vi "_PC_Daemon_Config_D999.vi"(8 "error in (no error)":errorcluster) -> (0 "error out":errorcluster)   [LabVIEW 2018]
uses:
  PublicSubVI/Ctl/RegistyFunc.ctl
  <resource>/objmgr/ni.var.rc
  <vilib>/Utility/miscctls.llb/LVBoundsTypeDef.ctl
panel:
  in  "Load":bool
  in  "Save":bool
  in  "Multiply":dbl[](array[numeric])=[1.0, 1.0, 1.0, 1.0, 1.0, 1.0, 1.0, 1.0, 1.0, 1.0, 1.0, 1.0]
  in  "Add":dbl[](array[numeric])=[0.0, 0.0, 0.0, 0.0, 0.0, 0.0, 0.0, 0.0, 0.0, 0.0, 0.0, 0.0]
  in  "Label":string[](array[string])=["", "", "", "", "", "", "", "", "", "", "", ""]
  in  "AI":string[](array[string])=["AI 0", "AI 1", "AI 2", "AI 3", "AI 4", "AI 5", "AI 6", "AI 7", "AI 8", "AI 9", "AI 10", "AI 11"]
  in  "AO":string[](array[string])=["AO 0", "AO 1", "AO 2", "AO 3", "AO 4", "AO 5", "AO 6", "AO 7", "AO 8"]
  in  "WriteValue":i16[](array[numeric])=[0, 0, 0, 0, 0, 0, 0, 0, 0] min=-4095 max=4095 step=1000
  in  "WriteColor":u32[](array[colorbox])=[16777224, 16777224, 16777224, 16777224, 16777224, 16777224, 16777224, 16777224, 16777224]
  in  "Scale":u16=1 min=1
  in  "Enable":bool
  in  "CEM(AO1)":bool
  in  "DYNODE(AO 0)":bool
  in  "ESPY(AO2)":bool
  in  "LENS(AO 3 : AO 8)":bool
  in  "Description":string="LENS : OFF; ESPY : OFF; DYNODE : OFF; CEN : OFF; "
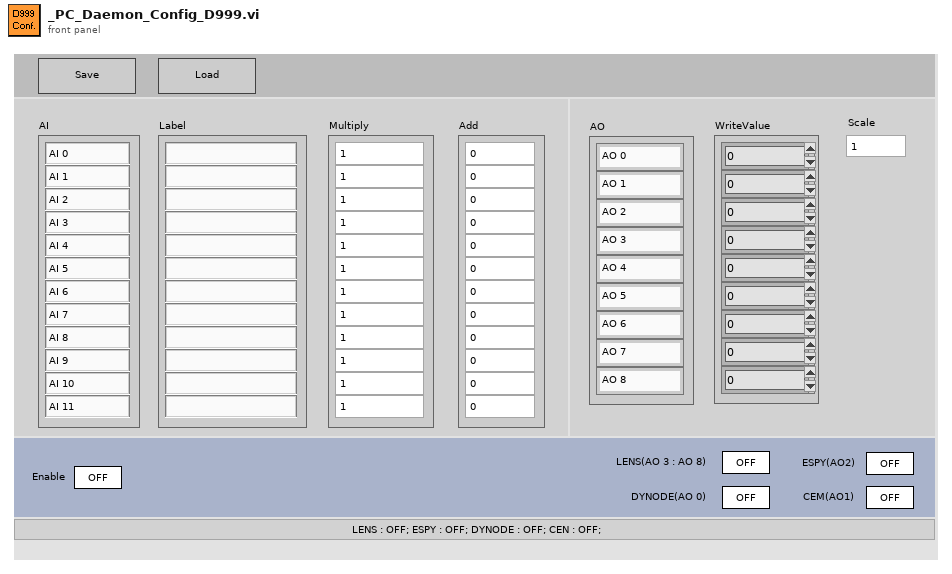
[diagram p1: front panel]
types:
  T1 = cluster{"Enable":refnum<vi>, "Label":refnum<vi>, "Multiply":refnum<vi>, "Add":refnum<vi>, "WriteColor":refnum<vi>, "WriteValue":refnum<vi>, "Description":refnum<vi>, "switch array":refnum<vi>[]}
  T2 = enum8{"Enabled", "Disabled", "Disabled and Grayed Out"}
  T3 = enum32{"Invalid", "Default", "Floating", "Floating/Auto-Hide", "Modal"}
  T4 = typedef "LVBoundsTypeDef.ctl" = cluster{"Width":u32, "Height":u32}
  T5 = cluster{"Label":string, "MultiValue":dbl, "AddValue":dbl}
  T6 = typedef "_ctl_RT_D999_Param.ctl" = cluster{"Enable":bool, "AI":cluster{"Label":string, "MultiValue":dbl, "AddValue":dbl}[], "AO":i16[], "Switch":bool[]}
  T7 = typedef "RegistyFunc.ctl" = enum16{"None", "FileAutoSave", "FileNoise", "FileSN", "ExeStatu", "WorkFolderPath", "MethodPath", "AVGItem", "LoopItem", "AutoRun", "BGColor", "LineColor", "LineWidth", "XGrid", "YGrid", "DeviceRefnum"}
  T8 = cluster{"Label":string[], "Multiply":dbl[], "Add":dbl[], "WriteValue":i16[], "switch":u32}
  T9 = typedef "eventvkey.ctl" = enum16{"ASCII", "Enter", "Return", "Shift", "Ctrl", "Alt", "Cmd", "Opt", "Caps", "NumLock", "Clear", "Break", "Up", "Down", "Left", "Right", "Insert", "Delete", "Home", "End", "PageUp", "PageDown", "Escape", "Help", "Pause", "ScrollLock", "F1", "F2", "F3", "F4", "F5", "F6", "F7", "F8", "F9", "F10", "F11", "F12", "F13", "F14", "F15", "F16", "F17", "F18", "F19", "F20", "F21", "F22", "F23", "F24", "Play", "VolumeUp", "VolumeDown", "Mute", "Two Byte Char"}
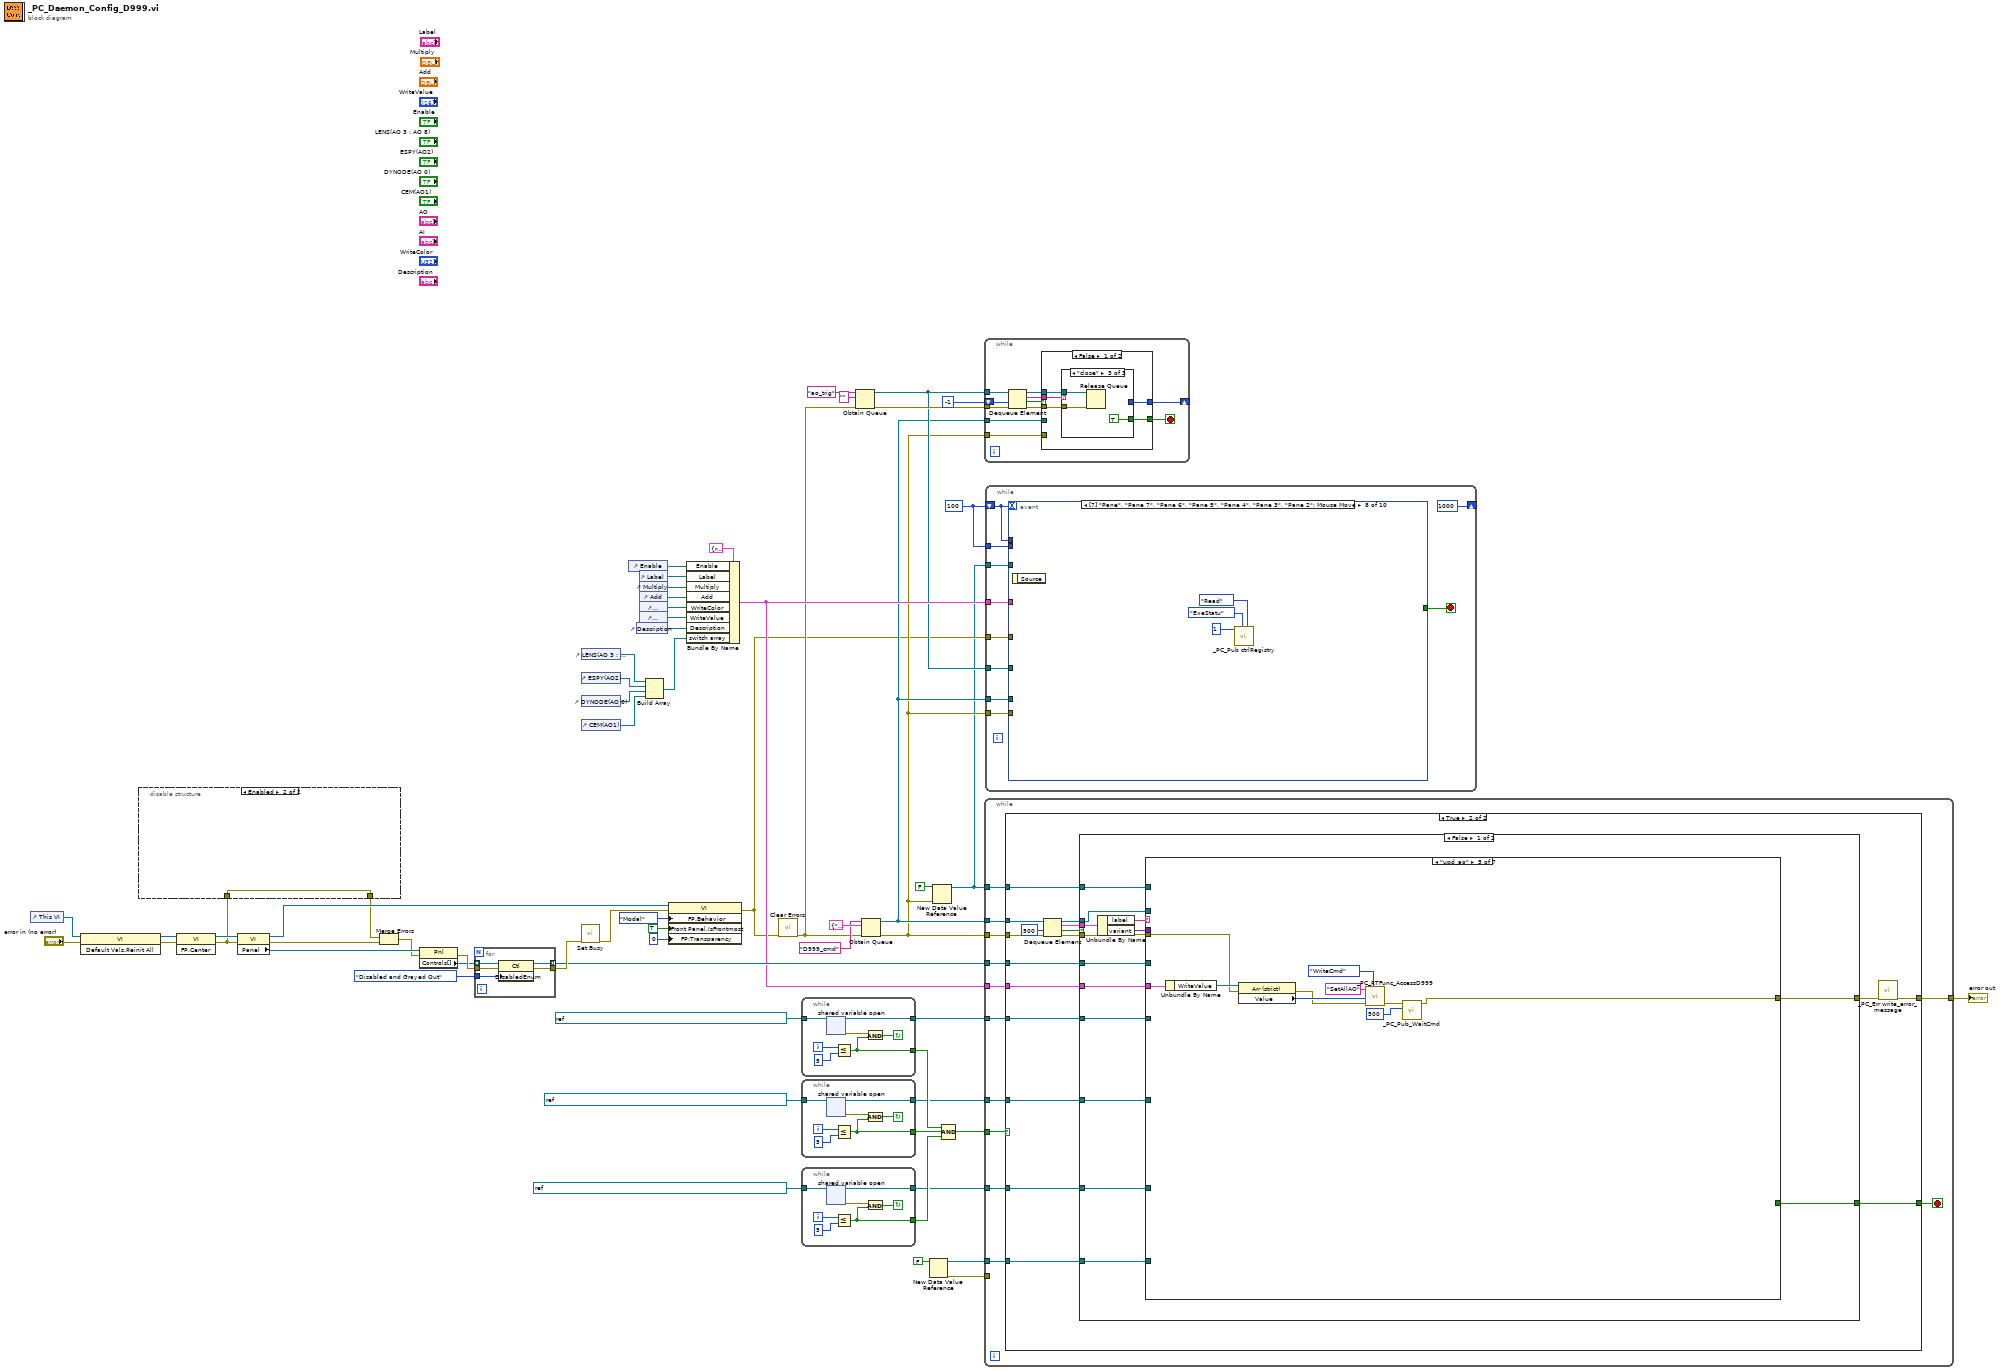
[diagram p0: block diagram]
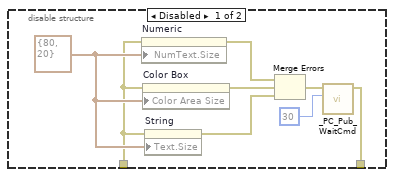
[diagram p2: hidden frame]
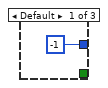
[diagram p3: hidden frame]
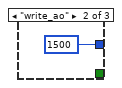
[diagram p4: hidden frame]
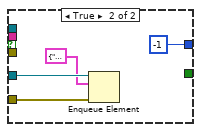
[diagram p5: hidden frame]
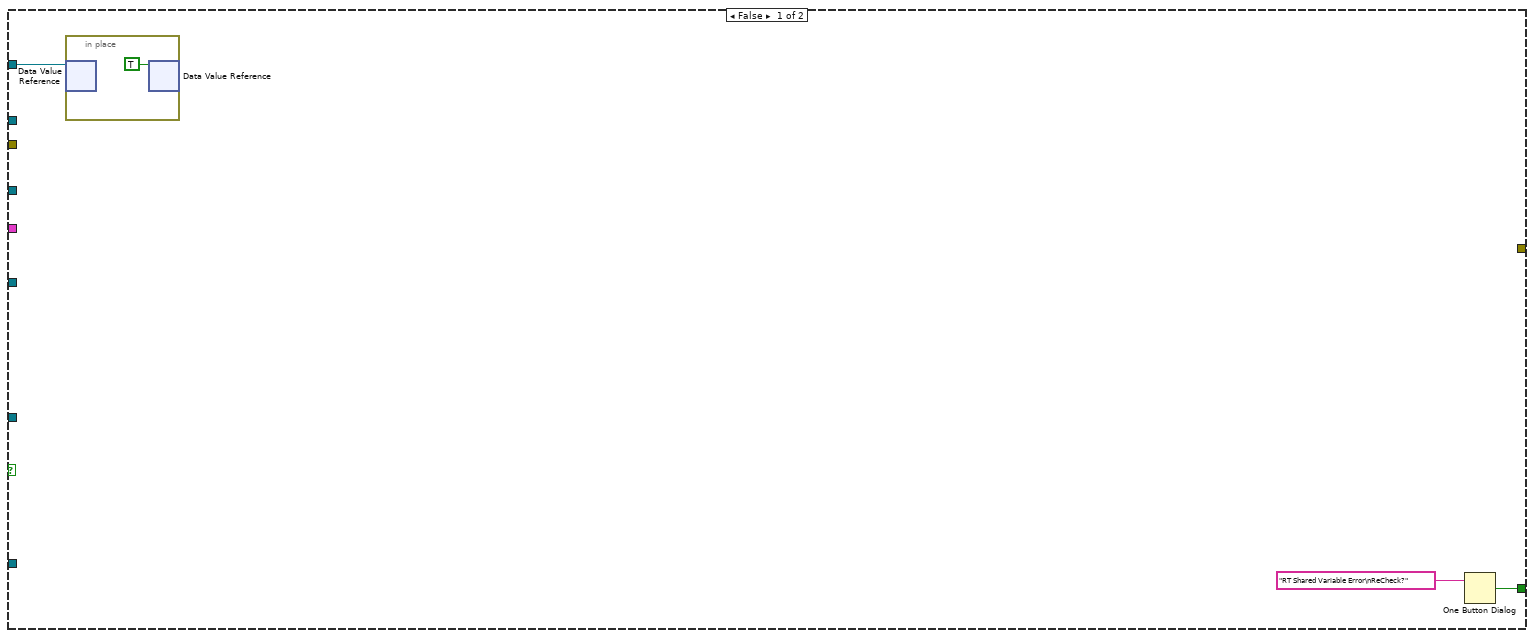
[diagram p6: hidden frame]
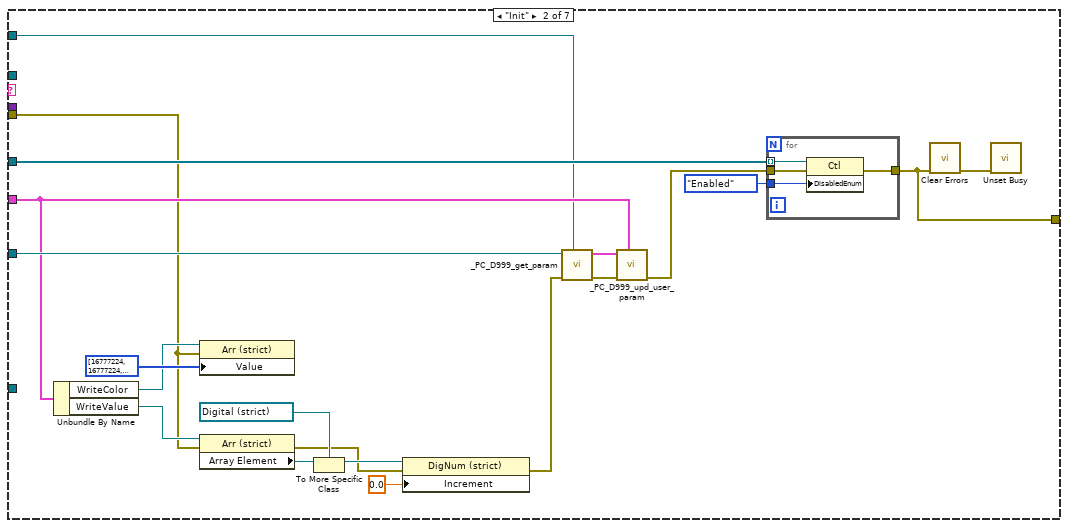
[diagram p8: hidden frame]
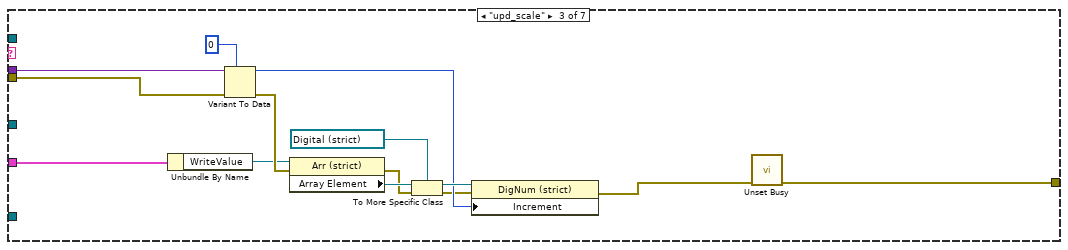
[diagram p9: hidden frame]
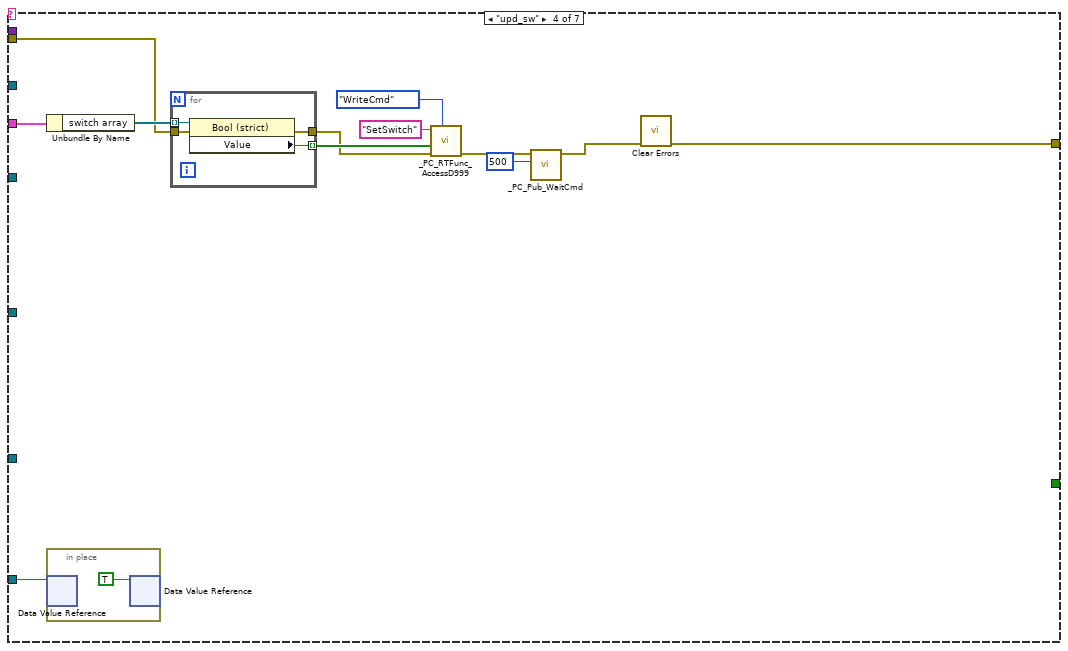
[diagram p10: hidden frame]
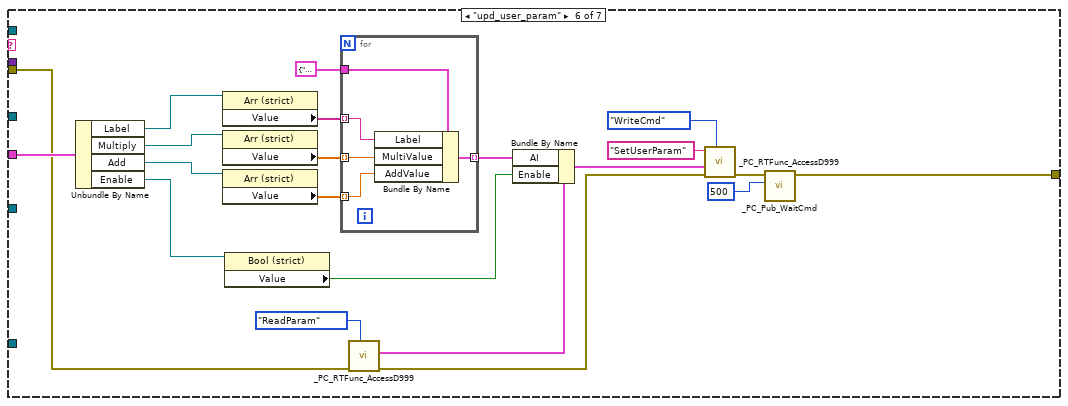
[diagram p11: hidden frame]
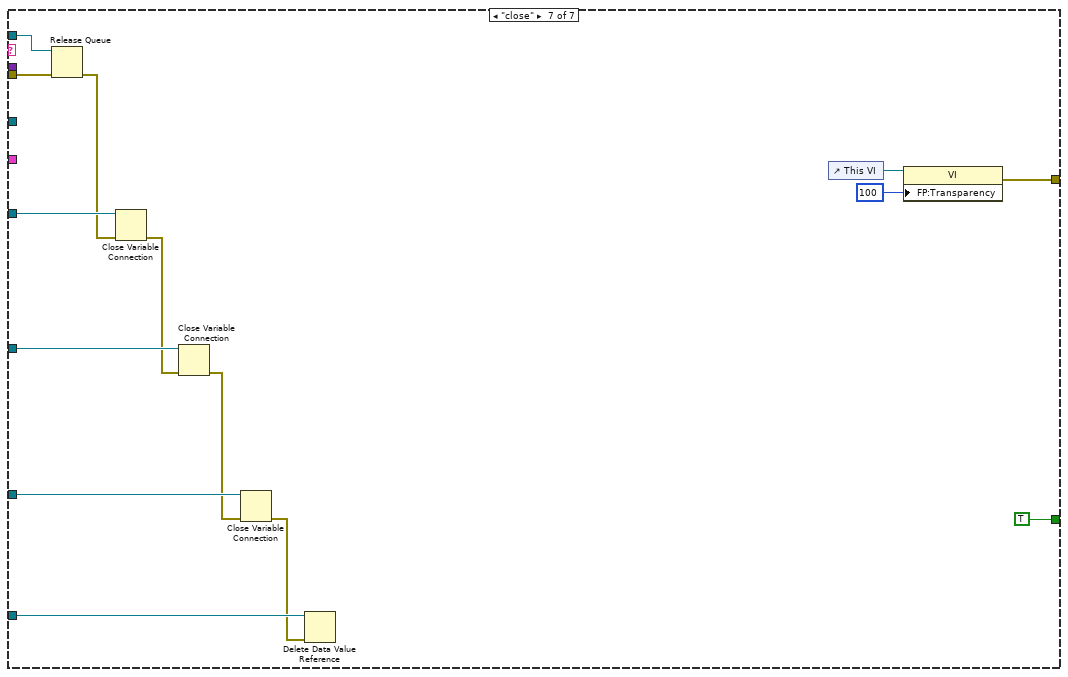
[diagram p12: hidden frame]
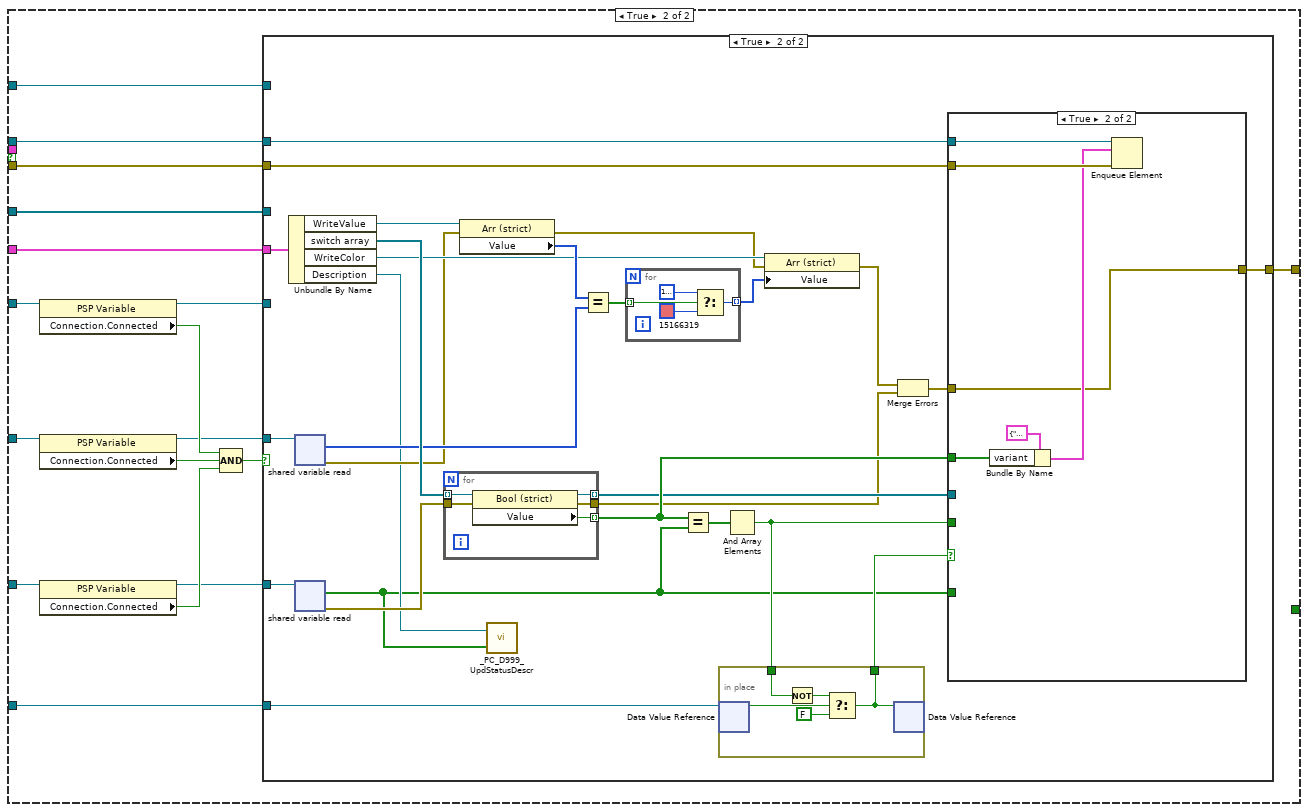
[diagram p13: hidden frame]
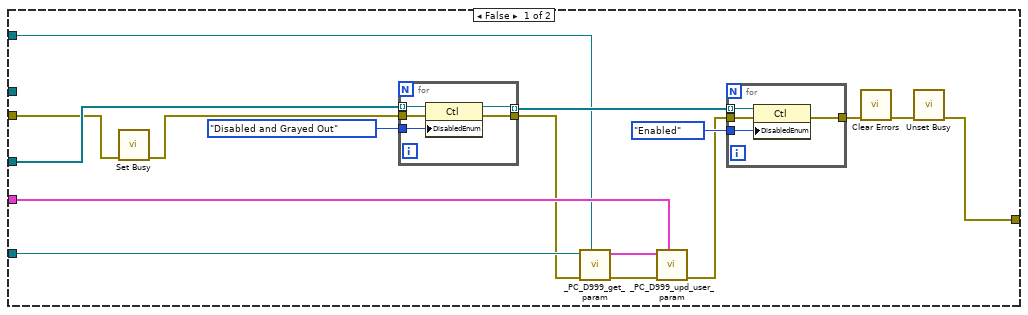
[diagram p14: hidden frame]
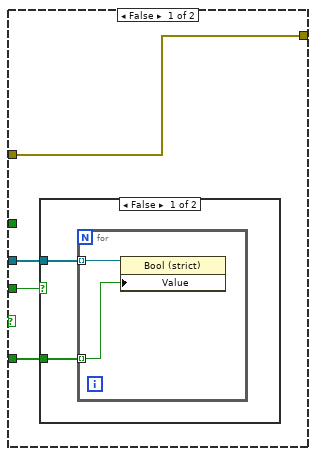
[diagram p15: hidden frame]
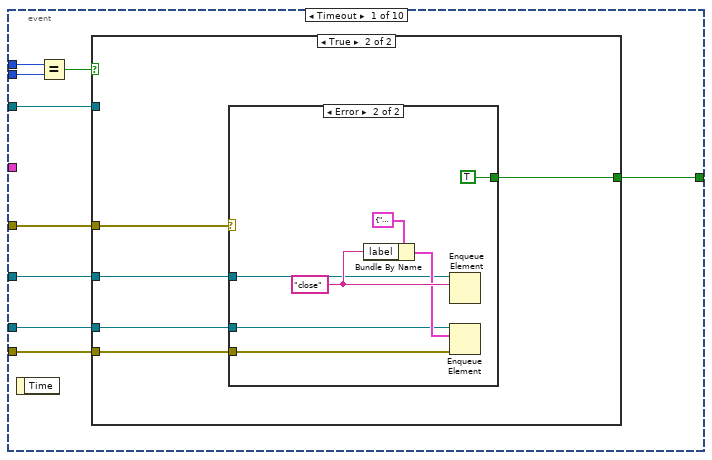
[diagram p17: hidden frame]
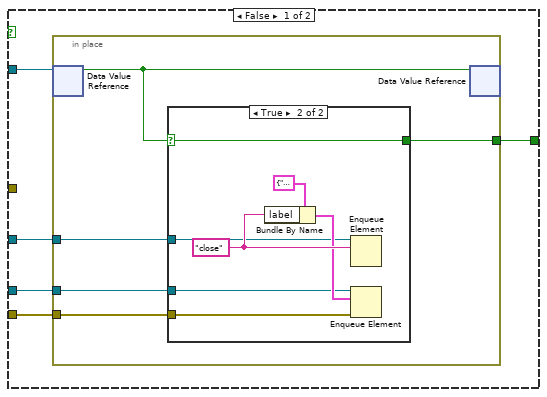
[diagram p18: hidden frame]
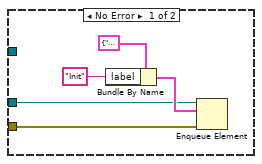
[diagram p20: hidden frame]
diagram:
  w2 = 100
  n1 = control-ref of="This VI"() -> (w59:refnum<vi>)
  n2 = invoke class="VI" method="Default Vals.Reinit All"(reference=w59, error in="error in (no error)") -> (reference out=w60:refnum<vi>, error out=w57:errorcluster)  [unwired: 1 in, 1 out]
  n3 = invoke class="VI" method="FP.Center"(reference=w60, error in=w57) -> (reference out=w52:refnum<vi>, error out=w9:errorcluster)  [unwired: 1 in, 1 out]
  n4 = disable-structure shown="Enabled" {
    disable-tunnel: w9 -> [w64 w71]
    disable-tunnel: [w63 w71] -> w6
    frame Disabled {
      w70 = T4 {"Width"=80, "Height"=20} ("Numeric Text.Size")
      n5 = property on="Numeric" class="DigNum (strict)"(error in=w64, "NumText.Size"=w70) -> (error out=w69:errorcluster)  [unwired: 1 in, 1 out]
      n6 = property on="Color Box" class="ColBox"(error in=w64, "Color Area Size"=w70) -> (error out=w68:errorcluster)  [unwired: 1 in, 1 out]
      n7 = property on="String" class="Str"(error in=w64, "Text.Size"=w70) -> (error out=w67:errorcluster)  [unwired: 1 in, 1 out]
      n8 = Merge Errors(w69, w68, w67) -> (w65:errorcluster)
      n9 = call "_PC_Pub_WaitCmd.vi"("milliseconds to wait"=u32 30, "error in (no error)"=w65) -> ("error out"=w63:errorcluster)  [unwired: 9 in]
    }
    frame Enabled {
    }
  }
  n10 = property class="VI"(reference=w52, error in=w9) -> (reference out=w51:refnum<vi>, error out=w7:errorcluster, "Panel"=w58:refnum<vi>)
  n11 = Merge Errors(w6, w7) -> (w5:errorcluster)
  n12 = property class="Pnl"(reference=w58, error in=w5) -> (error out=w55:errorcluster, "Controls[]"=w54:refnum<vi>[])  [unwired: 1 out]
  n13 = for {
    tunnel: w54 -> [w76] mode=indexing
    tunnel: T2."Disabled and Grayed Out" ("Disabled") -> [w75]
    tunnel: [w74] -> w23 mode=indexing
    tunnel: [w73] -> w50
    tunnel: w55 -> [w72]
    n14 = property class="Ctl"(reference=w76, error in=w72, "DisabledEnum"=w75) -> (reference out=w74:refnum<vi>, error out=w73:errorcluster)
  }
  n15 = control-ref of="LENS(AO 3 : AO 8)"() -> (w34:refnum<vi>)
  n16 = control-ref of="ESPY(AO2)"() -> (w35:refnum<vi>)
  n17 = control-ref of="DYNODE(AO 0)"() -> (w36:refnum<vi>)
  n18 = control-ref of="CEM(AO1)"() -> (w37:refnum<vi>)
  n19 = call <vilib>:"Set Busy.vi"("error in (no error)"=w50) -> ("error out"=w8:errorcluster)  [unwired: 9 in, 1 out]
  n20 = control-ref of="Enable"() -> (w32:refnum<vi>)
  n21 = control-ref of="Description"() -> (w26:refnum<vi>)
  n22 = control-ref of="Label"() -> (w31:refnum<vi>)
  n23 = control-ref of="Multiply"() -> (w30:refnum<vi>)
  n24 = control-ref of="Add"() -> (w29:refnum<vi>)
  n25 = control-ref of="WriteColor"() -> (w28:refnum<vi>)
  n26 = control-ref of="WriteValue"() -> (w27:refnum<vi>)
  n27 = Build Array(w34, w35, w36, w37) -> (w25:refnum<vi>[])
  n28 = property class="VI"(reference=w51, error in=w8, "FP.Behavior"=T3."Modal" ("Front Panel Window:Behavior"), "Front Panel.IsFrontmost"=TRUE ("Front Panel Window:Is Frontmost"), "FP:Transparency"=u8 0 ("Front Panel Window:Transparency")) -> (error out=w4:errorcluster)  [unwired: 1 out]
  n29 = Bundle By Name(cluster=T1 {"Enable"=refnum, "Label"=refnum, "Multiply"=refnum, "Add"=refnum, "WriteColor"=refnum, "WriteValue"=refnum, "Description"=refnum, "switch array"=[]}, "Enable"=w32, "Label"=w31, "Multiply"=w30, "Add"=w29, "WriteColor"=w28, "WriteValue"=w27, "Description"=w26, "switch array"=w25) -> (w20:T1)
  n30 = call <vilib>:"Clear Errors.vi"("error in (no error)"=w4) -> ("error out"=w17:errorcluster)  [unwired: 5 in, 1 out]
  n31 = while {
    tunnel: [w77] -> w45
    tunnel: refnum<k21> "ni.var.psp://NI-sbRIO/_RT_CtrlLoop_D999_Variables/D999_Exist" ("shared variable refnum in") -> [w83]
    tunnel: [w82] -> w46
    i -> [w80]
    stop <- w78 continue-if-true
    n32 = shared-variable-open(w83) -> (w82:refnum<k21>, w79:errorcluster)  [unwired: 1 in]
    n33 = Less Or Equal?(x=w80, y=5) -> (x <= y?=w77:bool)
    n34 = And(x=w79, y=w77) -> (x .and. y?=w78:bool)
  }
  n35 = while {
    tunnel: [w84] -> w44
    tunnel: refnum<k21> "ni.var.psp://NI-sbRIO/_RT_CtrlLoop_D999_Variables/D999_AO_Res" ("shared variable refnum in") -> [w90]
    tunnel: [w89] -> w39
    i -> [w87]
    stop <- w85 continue-if-true
    n36 = shared-variable-open(w90) -> (w89:refnum<k21>, w86:errorcluster)  [unwired: 1 in]
    n37 = Less Or Equal?(x=w87, y=5) -> (x <= y?=w84:bool)
    n38 = And(x=w86, y=w84) -> (x .and. y?=w85:bool)
  }
  n39 = while {
    tunnel: [w91] -> w43
    tunnel: refnum<k21> "ni.var.psp://NI-sbRIO/_RT_CtrlLoop_D999_Variables/D999_Switch_Res" ("shared variable refnum in") -> [w97]
    tunnel: [w96] -> w38
    i -> [w94]
    stop <- w92 continue-if-true
    n40 = shared-variable-open(w97) -> (w96:refnum<k21>, w93:errorcluster)  [unwired: 1 in]
    n41 = Less Or Equal?(x=w94, y=5) -> (x <= y?=w91:bool)
    n42 = And(x=w93, y=w91) -> (x .and. y?=w92:bool)
  }
  n43 = Obtain Queue(name (unnamed)="ao_trig", element data type="", error in (no error)=w17) -> (queue out=w16:refnum<queue>, error out=w18:errorcluster)  [unwired: 2 in, 1 out]
  n44 = Obtain Queue(name (unnamed)="D999_cmd", element data type=cluster{"label":string, "variant":variant} {"label"="", "variant"=variant}, error in (no error)=w17) -> (queue out=w13:refnum<queue>, error out=w10:errorcluster)  [unwired: 2 in, 1 out]
  n45 = New Data Value Reference(data value=FALSE) -> (data value reference=w24:refnum<data-value>, error out=w21:errorcluster)  [unwired: 1 in]
  n46 = New Data Value Reference(data value=FALSE, error in=w10) -> (data value reference=w1:refnum<data-value>)  [unwired: 1 out]
  n47 = Compound Arithmetic op=AND(w45, w44, w43) -> (w42:bool)
  n48 = while {
    tunnel: w16 -> [w108]
    tunnel: w18 -> [w106]
    shift-right: [w101] -> _
    shift-left: -1 ("timeout in ms (-1)") -> [w107]
    tunnel: w13 -> [w99]
    tunnel: w10 -> [w98]
    stop <- w100 stop-if-true
    n49 = Dequeue Element(queue=w108, timeout in ms (-1)=w107, error in (no error)=w106) -> (queue out=w102:refnum<queue>, element=w104:string, timed out?=w105:bool, error out=w103:errorcluster)
    n50 = case shown="False" w105 {
      tunnel: w104 -> [w113 _]
      tunnel: w103 -> [w112 _]
      tunnel: w102 -> [w109 _]
      tunnel: [w111 -1] -> w101
      tunnel: [w110 _] -> w100
      tunnel: w99 -> [_ w121]
      tunnel: w98 -> [_ w120]
      frame False {
        n51 = case shown="\"close\"" w113 {
          tunnel: w112 -> [_ _ w116]
          tunnel: [-1 1500 _] -> w111
          tunnel: [_ _ TRUE] -> w110
          tunnel: w109 -> [_ _ w117]
          frame Default {
          }
          frame "write_ao" {
          }
          frame "close" {
            n52 = Release Queue(queue=w117, error in (no error)=w116) -> ()  [unwired: 1 in, 3 out]
          }
        }
      }
      frame True {
        n53 = Enqueue Element(queue=w121, element=cluster{"label":string, "variant":variant} {"label"="upd_ao", "variant"=variant}, error in (no error)=w120) -> ()  [unwired: 1 in, 3 out]
      }
    }
  }
  n54 = while {
    tunnel: w13 -> [w134]
    tunnel: w10 -> [w133]
    tunnel: w46 -> [w132]
    tunnel: w42 -> [w130]
    tunnel: w39 -> [w129]
    tunnel: w38 -> [w128]
    tunnel: w20 -> [w127]
    tunnel: w24 -> [w126]
    tunnel: w23 -> [w125]
    tunnel: w21 -> [_]
    tunnel: [w124] -> w12
    tunnel: w1 -> [w123]
    stop <- w131 stop-if-true
    n55 = case shown="True" w130 {
      tunnel: w134 -> [_ w155]
      tunnel: w133 -> [_ w154]
      tunnel: w132 -> [_ w149]
      tunnel: [w136 w141] -> w131
      tunnel: w129 -> [_ w148]
      tunnel: w128 -> [_ w147]
      tunnel: w127 -> [_ w146]
      tunnel: w126 -> [_ w144]
      tunnel: w125 -> [_ w143]
      tunnel: [_ w140] -> w124
      tunnel: w123 -> [w135 w139]
      frame False {
        n56 = in-place {
          n57 = in-place-dvr #1(w135) -> ()  [unwired: 2 out]
          n58 = in-place-dvr #1(TRUE ("data value")) -> ()  [unwired: 2 out]
        }
        n59 = One Button Dialog(message="RT Shared Variable Error\nReCheck?") -> (true=w136:bool)  [unwired: 1 in]
      }
      frame True {
        n60 = Dequeue Element(queue=w155, timeout in ms (-1)=500, error in (no error)=w154) -> (queue out=w145:refnum<queue>, element=w150:cluster{"label":string, "variant":variant}, timed out?=w152:bool, error out=w151:errorcluster)
        n61 = case shown="False" w152 {
          tunnel: w151 -> [w161 w281]
          tunnel: w150 -> [w169 _]
          tunnel: w149 -> [w166 w292]
          tunnel: w148 -> [w165 w291]
          tunnel: w147 -> [w164 w290]
          tunnel: w146 -> [w162 w283]
          tunnel: w145 -> [w157 w282]
          tunnel: w144 -> [w160 w280]
          tunnel: w143 -> [w163 w278]
          tunnel: [w159 w277] -> w142
          tunnel: [w158 _] -> w141
          tunnel: w139 -> [w156 w276]
          frame False {
            n62 = Unbundle By Name(w169) -> ("label"=w168:string, "variant"=w167:variant)
            n63 = case shown="\"upd_ao\"" w168 {
              tunnel: w167 -> [_ _ w203 _ _ _ _]
              tunnel: w166 -> [_ w187 _ _ _ _ w272]
              tunnel: w165 -> [_ _ _ _ _ _ w270]
              tunnel: w164 -> [_ _ _ _ _ _ w268]
              tunnel: w163 -> [_ w190 _ _ _ _ _]
              tunnel: w162 -> [_ w183 w199 w215 w230 w244 _]
              tunnel: w161 -> [w170 w174 w195 w210 w228 w237 w273]
              tunnel: w160 -> [_ _ _ w212 _ _ w269]
              tunnel: [w170 w172 w196 w209 w226 w236 w262] -> w159
              tunnel: [_ _ _ _ _ _ TRUE] -> w158
              tunnel: w157 -> [_ _ _ _ _ _ w274]
              tunnel: w156 -> [_ w171 _ _ _ _ _]
              frame Default {
              }
              frame "Init" {
                n64 = Unbundle By Name(w183) -> ("WriteColor"=w175:refnum<vi>, "WriteValue"=w177:refnum<vi>)
                n65 = property class="Arr (strict)"(reference=w175, error in=w174, "Value"=u32[] [16777224, 16777224, 16777224, 16777224, 16777224, 16777224, 16777224, 16777224, 16777224]) -> ()  [unwired: 2 out]
                n66 = property class="Arr (strict)"(reference=w177, error in=w174) -> (error out=w178:errorcluster, "Array Element"=w182:refnum<vi>)  [unwired: 1 out]
                n67 = To More Specific Class(target class=refnum<vi> refnum ("Numeric"), reference=w182) -> (specific class reference=w179:refnum<vi>)  [unwired: 1 in, 1 out]
                n68 = property class="DigNum (strict)"(reference=w179, error in=w178, "Increment"=0.0 ("Data Entry Limits:Increment")) -> (error out=w173:errorcluster)  [unwired: 1 out]
                n69 = call "_PC_D999_get_param.vi"("stop cmd"=w171, "error in (no error)"=w173, "D999_exist SV"=w187) -> ("error out"=w188:errorcluster, "D999_Param"=w189:T6)  [unwired: 7 in]
                n70 = call "_PC_D999_upd_user_param.vi"("refnum cluster"=w183, "error in (no error)"=w188, "D999_Param"=w189) -> ("error out"=w186:errorcluster)  [unwired: 8 in]
                n71 = for {
                  tunnel: w190 -> [w194] mode=indexing
                  tunnel: T2."Enabled" ("Disabled") -> [w193]
                  tunnel: [w192] -> w172
                  tunnel: w186 -> [w191]
                  n72 = property class="Ctl"(reference=w194, error in=w191, "DisabledEnum"=w193) -> (error out=w192:errorcluster)  [unwired: 1 out]
                }
                n73 = call <vilib>:"Clear Errors.vi"("error in (no error)"=w172) -> ("error out"=w184:errorcluster)  [unwired: 5 in, 1 out]
                n74 = call <vilib>:"Unset Busy.vi"("error in (no error)"=w184) -> ()  [unwired: 10 in, 1 out]
              }
              frame "upd_scale" {
                n75 = Unbundle By Name(w199) -> ("WriteValue"=w198:refnum<vi>)
                n76 = Variant To Data(error in=w195, type=u16 0 ("NewVal"), Variant=w203) -> (data=w204:u16, error out=w200:errorcluster)
                n77 = property class="Arr (strict)"(reference=w198, error in=w200) -> (error out=w202:errorcluster, "Array Element"=w207:refnum<vi>)  [unwired: 1 out]
                n78 = To More Specific Class(target class=refnum<vi> refnum ("Numeric"), reference=w207, error in=w202) -> (specific class reference=w206:refnum<vi>, error out=w201:errorcluster)
                n79 = property class="DigNum (strict)"(reference=w206, error in=w201, "Increment"=w204) -> (error out=w197:errorcluster)  [unwired: 1 out]
                n80 = call <vilib>:"Unset Busy.vi"("error in (no error)"=w197) -> ("error out"=w196:errorcluster)  [unwired: 10 in]
              }
              frame "upd_sw" {
                n81 = Unbundle By Name(w215) -> ("switch array"=w214:refnum<vi>[])
                n82 = in-place {
                  n83 = in-place-dvr #2(w212) -> ()  [unwired: 2 out]
                  n84 = in-place-dvr #2(TRUE ("data value")) -> ()  [unwired: 2 out]
                }
                n85 = for {
                  tunnel: w214 -> [w225] mode=indexing
                  tunnel: [w224] -> w219 mode=indexing
                  tunnel: w210 -> [w223]
                  tunnel: [w222] -> w213
                  n86 = property class="Bool (strict)"(reference=w225, error in=w223) -> (error out=w222:errorcluster, "Value"=w224:bool)  [unwired: 1 out]
                }
                n87 = call "_PC_RTFunc_AccessD999.vi"("Function"=enum16{"WriteCmd", "ReadParam", "ReadResponse"}."WriteCmd", "error in (no error)"=w213, "Variant"=w219, "Cmd"="SetSwitch") -> ("error out"=w218:errorcluster)  [unwired: 6 in, 1 out]
                n88 = call "_PC_Pub_WaitCmd.vi"("milliseconds to wait"=u32 500, "error in (no error)"=w218) -> ("error out"=w211:errorcluster)  [unwired: 9 in]
                n89 = call <vilib>:"Clear Errors.vi"("error in (no error)"=w211) -> ("error out"=w209:errorcluster)  [unwired: 5 in, 1 out]
              }
              frame "upd_ao" {
                n90 = Unbundle By Name(w230) -> ("WriteValue"=w229:refnum<vi>)
                n91 = property class="Arr (strict)"(reference=w229, error in=w228) -> (error out=w227:errorcluster, "Value"=w234:i16[])  [unwired: 1 out]
                n92 = call "_PC_RTFunc_AccessD999.vi"("Function"=enum16{"WriteCmd", "ReadParam", "ReadResponse"}."WriteCmd", "error in (no error)"=w227, "Variant"=w234, "Cmd"="SetAllAO") -> ("error out"=w233:errorcluster)  [unwired: 6 in, 1 out]
                n93 = call "_PC_Pub_WaitCmd.vi"("milliseconds to wait"=u32 500, "error in (no error)"=w233) -> ("error out"=w226:errorcluster)  [unwired: 9 in]
              }
              frame "upd_user_param" {
                n94 = Unbundle By Name(w244) -> ("Label"=w243:refnum<vi>, "Multiply"=w242:refnum<vi>, "Add"=w241:refnum<vi>, "Enable"=w240:refnum<vi>)
                n95 = property class="Arr (strict)"(reference=w243) -> ("Value"=w253:string[])  [unwired: 1 in, 2 out]
                n96 = property class="Arr (strict)"(reference=w242) -> ("Value"=w252:dbl[])  [unwired: 1 in, 2 out]
                n97 = property class="Arr (strict)"(reference=w241) -> ("Value"=w251:dbl[])  [unwired: 1 in, 2 out]
                n98 = property class="Bool (strict)"(reference=w240) -> ("Value"=w248:bool)  [unwired: 1 in, 2 out]
                n99 = for {
                  tunnel: T5 {"Label"="", "MultiValue"=0.0, "AddValue"=0.0} ("EC_Param Cluster") -> [w261]
                  tunnel: w253 -> [w260] mode=indexing
                  tunnel: w252 -> [w259] mode=indexing
                  tunnel: w251 -> [w258] mode=indexing
                  tunnel: [w257] -> w250 mode=indexing
                  n100 = Bundle By Name(cluster=w261, "Label"=w260, "MultiValue"=w259, "AddValue"=w258) -> (w257:T5)
                }
                n101 = call "_PC_RTFunc_AccessD999.vi"("Function"=enum16{"WriteCmd", "ReadParam", "ReadResponse"}."ReadParam", "error in (no error)"=w237) -> ("error out"=w246:errorcluster, "D999_Param"=w249:T6)  [unwired: 8 in]
                n102 = Bundle By Name(cluster=w249, "AI"=w250, "Enable"=w248) -> (w247:T6)
                n103 = call "_PC_RTFunc_AccessD999.vi"("Function"=enum16{"WriteCmd", "ReadParam", "ReadResponse"}."WriteCmd", "error in (no error)"=w246, "Variant"=w247, "Cmd"="SetUserParam") -> ("error out"=w239:errorcluster)  [unwired: 6 in, 1 out]
                n104 = call "_PC_Pub_WaitCmd.vi"("milliseconds to wait"=u32 500, "error in (no error)"=w239) -> ("error out"=w236:errorcluster)  [unwired: 9 in]
              }
              frame "close" {
                n105 = Release Queue(queue=w274, error in (no error)=w273) -> (error out=w271:errorcluster)  [unwired: 1 in, 2 out]
                n106 = Close Variable Connection(8:w271, 11:w272) -> (0:w267:errorcluster)
                n107 = Close Variable Connection(8:w267, 11:w270) -> (0:w266:errorcluster)
                n108 = Close Variable Connection(8:w266, 11:w268) -> (0:w265:errorcluster)
                n109 = Delete Data Value Reference(data value reference=w269, error in=w265) -> ()  [unwired: 2 out]
                n110 = control-ref of="This VI"() -> (w264:refnum<vi>)
                n111 = property class="VI"(reference=w264, "FP:Transparency"=u8 100 ("Front Panel Window:Transparency")) -> (error out=w262:errorcluster)  [unwired: 1 in, 1 out]
              }
            }
          }
          frame True {
            n112 = property class="PSP Variable"(reference=w292) -> (reference out=w279:refnum<k21>, "Connection.Connected"=w288:bool)  [unwired: 1 in, 1 out]
            n113 = property class="PSP Variable"(reference=w291) -> (reference out=w285:refnum<k21>, "Connection.Connected"=w289:bool)  [unwired: 1 in, 1 out]
            n114 = property class="PSP Variable"(reference=w290) -> (reference out=w284:refnum<k21>, "Connection.Connected"=w287:bool)  [unwired: 1 in, 1 out]
            n115 = Compound Arithmetic op=AND(w288, w289, w287) -> (w286:bool)
            n116 = case shown="True" w286 {
              tunnel: w285 -> [_ w344]
              tunnel: w284 -> [_ w343]
              tunnel: w283 -> [w305 w342]
              tunnel: w282 -> [_ w327]
              tunnel: w281 -> [w296 w328]
              tunnel: w280 -> [_ w337]
              tunnel: w279 -> [w306 _]
              tunnel: w278 -> [w299 _]
              tunnel: [w294 w320] -> w277
              tunnel: w276 -> [w293 _]
              frame False {
                n117 = call <vilib>:"Set Busy.vi"("error in (no error)"=w296) -> ("error out"=w295:errorcluster)  [unwired: 9 in, 1 out]
                n118 = for {
                  tunnel: w299 -> [w313] mode=indexing
                  tunnel: T2."Disabled and Grayed Out" ("Disabled") -> [w312]
                  tunnel: [w311] -> w297
                  tunnel: w295 -> [w310]
                  tunnel: [w309] -> w298 mode=indexing
                  n119 = property class="Ctl"(reference=w313, error in=w310, "DisabledEnum"=w312) -> (reference out=w309:refnum<vi>, error out=w311:errorcluster)
                }
                n120 = call "_PC_D999_get_param.vi"("stop cmd"=w293, "error in (no error)"=w297, "D999_exist SV"=w306) -> ("error out"=w307:errorcluster, "D999_Param"=w308:T6)  [unwired: 7 in]
                n121 = call "_PC_D999_upd_user_param.vi"("refnum cluster"=w305, "error in (no error)"=w307, "D999_Param"=w308) -> ("error out"=w301:errorcluster)  [unwired: 8 in]
                n122 = for {
                  tunnel: w298 -> [w317] mode=indexing
                  tunnel: T2."Enabled" ("Disabled") -> [w316]
                  tunnel: [w315] -> w302
                  tunnel: w301 -> [w314]
                  n123 = property class="Ctl"(reference=w317, error in=w314, "DisabledEnum"=w316) -> (error out=w315:errorcluster)  [unwired: 1 out]
                }
                n124 = call <vilib>:"Clear Errors.vi"("error in (no error)"=w302) -> ("error out"=w303:errorcluster)  [unwired: 5 in, 1 out]
                n125 = call <vilib>:"Unset Busy.vi"("error in (no error)"=w303) -> ("error out"=w294:errorcluster)  [unwired: 10 in]
              }
              frame True {
                n126 = Unbundle By Name(w342) -> ("WriteValue"=w340:refnum<vi>, "switch array"=w341:refnum<vi>[], "WriteColor"=w330:refnum<vi>, "Description"=w319:refnum<vi>)
                n127 = shared-variable-read(w344) -> (w326:errorcluster, w339:i16[])  [unwired: 1 in, 1 out]
                n128 = shared-variable-read(w343) -> (w324:errorcluster, w318:bool[])  [unwired: 1 in, 1 out]
                n129 = for {
                  tunnel: w341 -> [w372] mode=indexing
                  tunnel: [w371] -> w335 mode=indexing
                  tunnel: [w370] -> w332 mode=indexing
                  tunnel: w324 -> [w369]
                  tunnel: [w368] -> w322
                  n130 = property class="Bool (strict)"(reference=w372, error in=w369) -> (reference out=w370:refnum<vi>, error out=w368:errorcluster, "Value"=w371:bool)
                }
                n131 = property class="Arr (strict)"(reference=w340, error in=w326) -> (error out=w325:errorcluster, "Value"=w334:i16[])  [unwired: 1 out]
                n132 = call "_PC_D999_UpdStatusDescr.vi"("Switch Enable"=w318, "Description"=w319) -> ()  [unwired: 1 in]
                n133 = Equal?(x=w334, y=w339) -> (x = y?=w329:bool[])
                n134 = for {
                  tunnel: w329 -> [w348] mode=indexing
                  tunnel: [w345] -> w331 mode=indexing
                  n135 = Select(t=u32 16777224, s=w348, f=u32 15166319) -> (s? t:f=w345:u32)
                }
                n136 = Equal?(x=w335, y=w318) -> (x = y?=w338:bool[])
                n137 = And Array Elements(Boolean array=w338) -> (logical AND=w333:bool)
                n138 = in-place {
                  in-place-border: w333 -> [w366]
                  in-place-border: [w363] -> w336
                  n139 = in-place-dvr #3(w337) -> (w367:bool)  [unwired: 1 out]
                  n140 = Not(x=w366) -> (.not. x?=w365:bool)
                  n141 = Select(t=w365, s=w367, f=FALSE) -> (s? t:f=w363:bool)
                  n142 = in-place-dvr #3(w363) -> ()  [unwired: 2 out]
                }
                n143 = property class="Arr (strict)"(reference=w330, error in=w325, "Value"=w331) -> (error out=w323:errorcluster)  [unwired: 1 out]
                n144 = Merge Errors(w323, w322) -> (w321:errorcluster)
                n145 = case shown="True" w336 {
                  tunnel: w327 -> [_ w362]
                  tunnel: w328 -> [_ w361]
                  tunnel: w335 -> [_ w359]
                  tunnel: w333 -> [w351 _]
                  tunnel: w332 -> [w352 _]
                  tunnel: w318 -> [w350 _]
                  tunnel: w321 -> [w349 w357]
                  tunnel: [w349 w357] -> w320
                  frame False {
                    n146 = case shown="False" w351 {
                      tunnel: w352 -> [w354 _]
                      tunnel: w350 -> [w353 _]
                      frame False {
                        n147 = for {
                          tunnel: w354 -> [w356] mode=indexing
                          tunnel: w353 -> [w355] mode=indexing
                          n148 = property class="Bool (strict)"(reference=w356, "Value"=w355) -> ()  [unwired: 1 in, 2 out]
                        }
                      }
                      frame True {
                      }
                    }
                  }
                  frame True {
                    n149 = Bundle By Name(cluster=cluster{"label":string, "variant":variant} {"label"="upd_sw", "variant"=variant} ("element"), "variant"=w359) -> (w358:cluster{"label":string, "variant":variant})
                    n150 = Enqueue Element(queue=w362, element=w358, error in (no error)=w361) -> ()  [unwired: 1 in, 3 out]
                  }
                }
              }
            }
          }
        }
        n151 = call "_PC_Err write_error_message.vi"("error in"=w142) -> ("error out"=w140:errorcluster)  [unwired: 10 in]
      }
    }
  }
  "error out" <- w12
  n152 = while {
    tunnel: w20 -> [w382]
    shift-right: [1000] -> _
    shift-left: w2 -> [w375]
    tunnel: w4 -> [w379]
    tunnel: w13 -> [w378]
    tunnel: w10 -> [w377]
    tunnel: w16 -> [w376]
    tunnel: w2 -> [w374]
    tunnel: w1 -> [w373]
    stop <- w381 stop-if-true
    n153 = event shown="[7] \"Pane\", \"Pane 7\", \"Pane 6\", \"Pane 5\", \"Pane 4\", \"Pane 3\", \"Pane 2\": Mouse Move" {
      selector: _ -> [_ _ _ _ _ _ _ _ _ _]
      dyn-events: _ -> [_ _ _ _ _ _ _ _ _ _]
      timeout: w375 -> [_ _ _ _ _ _ _ _ _ _]
      tunnel: [w391 _ _ _ _ _ _ _ TRUE w503] -> w381
      tunnel: w382 -> [_ w429 w436 _ _ _ _ _ _ _]
      tunnel: w379 -> [w390 _ _ _ _ _ _ _ _ _]
      tunnel: w378 -> [w389 _ w432 w452 w455 _ w485 _ w493 w500]
      tunnel: w377 -> [w388 _ w431 w453 w454 w467 w481 _ w491 w499]
      tunnel: w376 -> [w387 _ _ _ _ w469 _ _ w494 w501]
      tunnel: w375 -> [w386 _ _ _ _ _ _ _ _ _]
      tunnel: w374 -> [w385 _ _ _ _ _ _ _ _ _]
      tunnel: w373 -> [w383 _ _ _ _ _ _ _ _ _]
      event Timeout {
        n154 = event-data() -> ()  [unwired: 1 in, 1 out]
        n155 = Equal?(x=w386, y=w385) -> (x = y?=w384:bool)
        n156 = case shown="True" w384 {
          tunnel: [w392 w414] -> w391
          tunnel: w390 -> [_ w413]
          tunnel: w389 -> [w394 w412]
          tunnel: w388 -> [w393 w411]
          tunnel: w387 -> [w395 w410]
          tunnel: w383 -> [w396 _]
          frame False {
            n157 = in-place {
              in-place-border: w395 -> [w399]
              in-place-border: w394 -> [w400]
              in-place-border: w393 -> [w401]
              in-place-border: [w397] -> w392
              n158 = in-place-dvr #4(w396) -> (w398:bool)  [unwired: 1 out]
              n159 = case shown="True" w398 {
                selector: w398 -> [w402 w403]
                tunnel: w401 -> [_ w406]
                tunnel: w400 -> [_ w405]
                tunnel: w399 -> [_ w404]
                tunnel: [w402 w403] -> w397
                frame False {
                }
                frame True {
                  w408 = "close" ("element")
                  n160 = Bundle By Name(cluster=cluster{"label":string, "variant":variant} {"label"="", "variant"=variant} ("element"), "label"=w408) -> (w407:cluster{"label":string, "variant":variant})
                  n161 = Enqueue Element(queue=w404, element=w408) -> ()  [unwired: 2 in, 3 out]
                  n162 = Enqueue Element(queue=w405, element=w407, error in (no error)=w406) -> ()  [unwired: 1 in, 3 out]
                }
              }
              n163 = in-place-dvr #4(w398) -> ()  [unwired: 2 out]
            }
          }
          frame True {
            n164 = case shown="Error" w413 {
              tunnel: [_ TRUE ("true")] -> w414
              tunnel: w412 -> [w416 w421]
              tunnel: w411 -> [w415 w420]
              tunnel: w410 -> [_ w422]
              frame No Error {
                n165 = Bundle By Name(cluster=cluster{"label":string, "variant":variant} {"label"="", "variant"=variant} ("element"), "label"="Init") -> (w417:cluster{"label":string, "variant":variant})
                n166 = Enqueue Element(queue=w416, element=w417, error in (no error)=w415) -> ()  [unwired: 1 in, 3 out]
              }
              frame Error {
                w424 = "close" ("element")
                n167 = Bundle By Name(cluster=cluster{"label":string, "variant":variant} {"label"="", "variant"=variant} ("element"), "label"=w424) -> (w423:cluster{"label":string, "variant":variant})
                n168 = Enqueue Element(queue=w422, element=w424) -> ()  [unwired: 2 in, 3 out]
                n169 = Enqueue Element(queue=w421, element=w423, error in (no error)=w420) -> ()  [unwired: 1 in, 3 out]
              }
            }
          }
        }
      }
      event "Save": Value Change {
        n170 = event-data() -> ()  [unwired: 1 in, 1 out]
        n171 = call "_PC_D999 config_param.vi"("Enum"=enum8{"None", "Write", "Read"}."Write", "Refnum cluster in"=w429) -> ("error out"=w427:errorcluster)  [unwired: 7 in, 2 out]
        n172 = case shown="Error" w427 {
          frame No Error {
          }
          frame Error {
            n173 = One Button Dialog(message="Save Failure") -> ()  [unwired: 1 in, 1 out]
          }
        }
      }
      event "Load": Value Change {
        n174 = event-data() -> ()  [unwired: 1 in, 1 out]
        n175 = call "_PC_D999 config_param.vi"("Enum"=enum8{"None", "Write", "Read"}."Read", "Refnum cluster in"=w436) -> ("error out"=w435:errorcluster, "data cluster output"=w433:T8, "Refnum cluster out"=w434:T1)  [unwired: 7 in]
        n176 = case shown="No Error" w435 {
          tunnel: w434 -> [w449 _]
          tunnel: w433 -> [w448 _]
          tunnel: w432 -> [w447 _]
          tunnel: w431 -> [w438 _]
          frame No Error {
            n177 = call "_PC_D999 data_collapse.vi"("error in (no error)"=w438, "data cluster in"=w448, "Refnum cluster in"=w449) -> ("error out"=w439:errorcluster)  [unwired: 7 in, 1 out]
            n178 = Enqueue Element(queue=w447, element=cluster{"label":string, "variant":variant} {"label"="upd_user_param", "variant"=variant}, error in (no error)=w439) -> (queue out=w445:refnum<queue>, error out=w446:errorcluster)  [unwired: 1 in, 1 out]
            n179 = Enqueue Element(queue=w445, element=cluster{"label":string, "variant":variant} {"label"="upd_ao", "variant"=variant}, error in (no error)=w446) -> (queue out=w444:refnum<queue>, error out=w443:errorcluster)  [unwired: 1 in, 1 out]
            n180 = Enqueue Element(queue=w444, element=cluster{"label":string, "variant":variant} {"label"="upd_sw", "variant"=variant}, error in (no error)=w443) -> ()  [unwired: 1 in, 3 out]
          }
          frame Error {
            n181 = One Button Dialog(message="Load Failure") -> ()  [unwired: 1 in, 1 out]
          }
        }
      }
      event "LENS(AO 3 : AO 8)", "ESPY(AO2)", "DYNODE(AO 0)", "CEM(AO1)": Value Change {
        n182 = event-data() -> ()  [unwired: 1 in, 1 out]
        n183 = Enqueue Element(queue=w452, element=cluster{"label":string, "variant":variant} {"label"="upd_sw", "variant"=variant}, error in (no error)=w453) -> ()  [unwired: 1 in, 3 out]
      }
      event "Enable": Value Change {
        n184 = event-data() -> ()  [unwired: 1 in, 6 out]
        n185 = Enqueue Element(queue=w455, element=cluster{"label":string, "variant":variant} {"label"="upd_user_param", "variant"=variant}, error in (no error)=w454) -> ()  [unwired: 1 in, 3 out]
      }
      event "WriteValue": Value Change {
        n186 = event-data() -> ("CtlRef"=w466:refnum<vi>, "OldVal"=w465:i16[], "NewVal"=w458:i16[])  [unwired: 1 in]
        n187 = Not Equal?(x=w465, y=w458) -> (x != y?=w464:bool[])
        n188 = Enqueue Element(queue=w469, element="write_ao" ("label"), error in (no error)=w467) -> ()  [unwired: 1 in, 3 out]
        n189 = Search 1D Array(1D array=w464, element=TRUE) -> (index of element=w457:i32)  [unwired: 1 in]
        n190 = Less?(x=w457, y=3) -> (x < y?=w460:bool)
        n191 = Greater Or Equal To 0?(x=w457) -> (x >= 0?=w461:bool)
        n192 = And(x=w461, y=w460) -> (x .and. y?=w459:bool)
        n193 = case shown="True" w459 {
          tunnel: w466 -> [_ w474]
          tunnel: w458 -> [_ w473]
          tunnel: w457 -> [_ w472]
          frame False {
          }
          frame True {
            n194 = Index Array(array=w473, index=w472) -> (element=w471:i16)
            n195 = Less Than 0?(x=w471) -> (x < 0?=w470:bool)
            n196 = case shown="True" w470 {
              tunnel: w474 -> [_ w479]
              tunnel: w473 -> [_ w476]
              tunnel: w472 -> [_ w475]
              frame False {
              }
              frame True {
                n197 = Replace Array Subset(array=w476, new element=i16 0 ("new element/subarray"), index=w475) -> (w477:i16[])
                n198 = property class="Arr (strict)"(reference=w479, "Value"=w477) -> ()  [unwired: 1 in, 2 out]
              }
            }
          }
        }
      }
      event "Scale": Value Change {
        n199 = event-data() -> ("NewVal"=w483:u16)  [unwired: 1 in]
        n200 = call <vilib>:"Set Busy.vi"("error in (no error)"=w481) -> ("error out"=w480:errorcluster)  [unwired: 9 in, 1 out]
        n201 = Bundle By Name(cluster=cluster{"label":string, "variant":variant} {"label"="upd_scale", "variant"=variant}, "variant"=w483) -> (w482:cluster{"label":string, "variant":variant})
        n202 = Enqueue Element(queue=w485, element=w482, error in (no error)=w480) -> ()  [unwired: 1 in, 3 out]
      }
      event Mouse Move {
        n203 = event-data() -> ()  [unwired: 1 in, 1 out]
        n204 = call "_PC_Pub ctrlRegistry.vi"("type"=enum16{"None", "Write", "Read"}."Read", "function"=RegistyFunc."ExeStatu", "write value"=1) -> ()  [unwired: 5 in, 4 out]
      }
      event Panel Close {
        w496 = "close" ("element")
        n205 = event-data() -> ()  [unwired: 1 in, 1 out]
        n206 = Enqueue Element(queue=w493, element=cluster{"label":string, "variant":variant} {"label"="upd_user_param", "variant"=variant}, error in (no error)=w491) -> (queue out=w492:refnum<queue>, error out=w489:errorcluster)  [unwired: 1 in, 1 out]
        n207 = Bundle By Name(cluster=cluster{"label":string, "variant":variant} {"label"="", "variant"=variant} ("element"), "label"=w496) -> (w495:cluster{"label":string, "variant":variant})
        n208 = Enqueue Element(queue=w494, element=w496, error in (no error)=w489) -> ()  [unwired: 1 in, 3 out]
        n209 = Enqueue Element(queue=w492, element=w495, error in (no error)=w489) -> ()  [unwired: 1 in, 3 out]
      }
      event Key Down? {
        n210 = event-data() -> ("VKey"=w502:T9)  [unwired: 1 in]
        n211 = case shown="\"Escape\"" w502 {
          tunnel: [_ TRUE] -> w503
          tunnel: w501 -> [_ w506]
          tunnel: w500 -> [_ w505]
          tunnel: w499 -> [_ w504]
          frame "ASCII", Default {
          }
          frame "Escape" {
            w511 = "close" ("element")
            n212 = Enqueue Element(queue=w505, element=cluster{"label":string, "variant":variant} {"label"="upd_user_param", "variant"=variant}, error in (no error)=w504) -> (queue out=w509:refnum<queue>, error out=w507:errorcluster)  [unwired: 1 in, 1 out]
            n213 = Bundle By Name(cluster=cluster{"label":string, "variant":variant} {"label"="", "variant"=variant} ("element"), "label"=w511) -> (w510:cluster{"label":string, "variant":variant})
            n214 = Enqueue Element(queue=w506, element=w511, error in (no error)=w507) -> ()  [unwired: 1 in, 3 out]
            n215 = Enqueue Element(queue=w509, element=w510, error in (no error)=w507) -> ()  [unwired: 1 in, 3 out]
          }
        }
        n216 = event-data("Discard?"=w503) -> ()  [unwired: 1 in, 1 out]
      }
    }
  }
